vi "change controller address.vi"() -> ()   [LabVIEW 2015]
panel:
  out "Controller ID# Found":u8
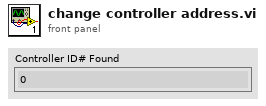
[diagram p1: front panel]
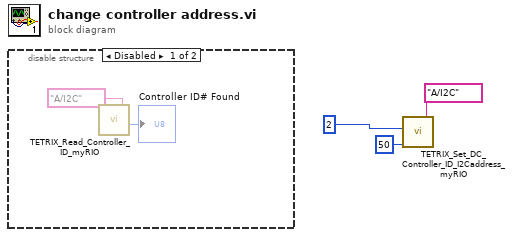
[diagram p0: block diagram]
diagram:
  n1 = disable-structure shown="Disabled" {
    frame Disabled {
      n2 = call <vilib>:"TETRIX_Read_Controller_ID_myRIO.vi"("myRIO MXP Port A/B"=tag "A/I2C") -> ("Controller ID# Found"=→"Controller ID# Found":u8)  [unwired: 5 in, 1 out]
    }
    frame Enabled {
    }
  }
  n3 = call <vilib>:"TETRIX_Set_DC_Controller_ID_I2Caddress_myRIO.vi"("myRIO MXP Port A/B"=tag "A/I2C", "New ID# / I2C Address"=u8 50, "Current ID#  / I2C Address"=u8 2) -> ()  [unwired: 4 in, 1 out]
